vi "ADSR_RT.vi"() -> ()   [LabVIEW 2014]
uses:
  Controls/ADSR State.ctl
  <vilib>/myRIO/Instrument Drivers/Onboard IO/AudioOut Block/typedefs/AudioOut Block Reference.ctl
  <vilib>/myRIO/Common/Instrument Driver Framework/Utilities/typedefs/myRIO Generic Hardware Reference.ctl
  <vilib>/myRIO/Common/Instrument Driver Framework/Utilities/typedefs/Hardware Version Enum.ctl
  <vilib>/myRIO/Common/Instrument Driver Framework/Utilities/typedefs/myRIO v1.0 Reference.ctl
  <vilib>/myRIO/Common/Instrument Driver Framework/Utilities/typedefs/Generic FPGA Reference.ctl
  <vilib>/myRIO/Common/Instrument Driver Framework/myRIO v1.0/AudioOut Block/typedefs/AudioOut Block Channels List.ctl
  <vilib>/myRIO/Common/Instrument Driver Framework/myRIO v1.0/AudioOut Block/typedefs/AudioOut Block Channels Enum.ctl
  <vilib>/myRIO/Common/Instrument Driver Framework/Utilities/typedefs/Analog Scaling Constants.ctl
  <vilib>/userdefined/High Color/nirio_resource_hc.ctl
  <vilib>/myRIO/Common/Instrument Driver Framework/Utilities/vis/Is FPGA Ref Available.vi
  <vilib>/myRIO/Common/Instrument Driver Framework/myRIO v1.0/AudioOut Block/vis/myRIO v1.1 Open Throughput AudioOut (N Samples).vi
  <vilib>/myRIO/Instrument Drivers/Onboard IO/AudioOut Block/vis/Write.vi
  <vilib>/myRIO/Common/Instrument Driver Framework/Utilities/vis/Validate Channels.vi
  <vilib>/Utility/VariantDataType/GetNumericInfo.vi
  <vilib>/Utility/error.llb/Error Cluster From Error Code.vi
  <vilib>/myRIO/Common/Instrument Driver Framework/myRIO v1.0/myRIO v1.1 Open Throughput.vi
  <vilib>/myRIO/Common/Instrument Driver Framework/myRIO v1.0/AudioOut Block/vis/myRIO v1.0 Get Scaling Constants AudioOut Block.vi
  <vilib>/myRIO/Common/Instrument Driver Framework/myRIO v1.0/AudioOut Block/vis/myRIO v1.0 Reserve AudioOut Block.vi
  <vilib>/myRIO/Common/Instrument Driver Framework/myRIO v1.0/Resource Manager/vis/myRIO v1.0 Open Writing DMA.vi
  <vilib>/myRIO/Common/Instrument Driver Framework/myRIO v1.0/myRIO v1.0 Close.vi
  <vilib>/myRIO/Common/Instrument Driver Framework/myRIO v1.0/AudioOut Block/vis/myRIO v1.0 AudioOut Block Write.vi
  <vilib>/myRIO/Express VI/Onboard IO/AudioOut/AudioOut Express VI.xnode
  <vilib>/myRIO/Instrument Drivers/Onboard IO/AudioOut Block/vis/myRIO AudioOut N Samples Open.xnode
  <vilib>/myRIO/Instrument Drivers/Onboard IO/AudioOut Block/AudioOut Block.lvlib
  <vilib>/measure/NI_MABase.lvlib
panel:
  in  "Stop Button":bool
  in  "Activate 2":bool
  out "f":T1
  out "Gain Graph 2":dbl(graph)
  out "Gain2":dbl
  in  "Release":dbl=300.0
  in  "Sustain 2":dbl=300.0
  in  "Decay (ms) 2":dbl=300.0
  in  "Sustain  2":dbl=60.0
  in  "Max. Amplitude (V) 2":dbl(slide)=0.7993311036789298 scale=0.0..1.0
  in  "Attack (ms) 2":dbl=1000.0
  in  "sampling info":cluster{"Fs":dbl, "#s":dbl}={"Fs"=10000.0, "#s"=1000.0} {"Fs" format="%.2p"}
  in  "Pitch Frequency":dbl=2200.0 format="%#_13g"
  out "End of Idle":i32=1002
  out "End":bool
  out "error out":errorcluster
  out "Waveform Chart":dbl[](graph)
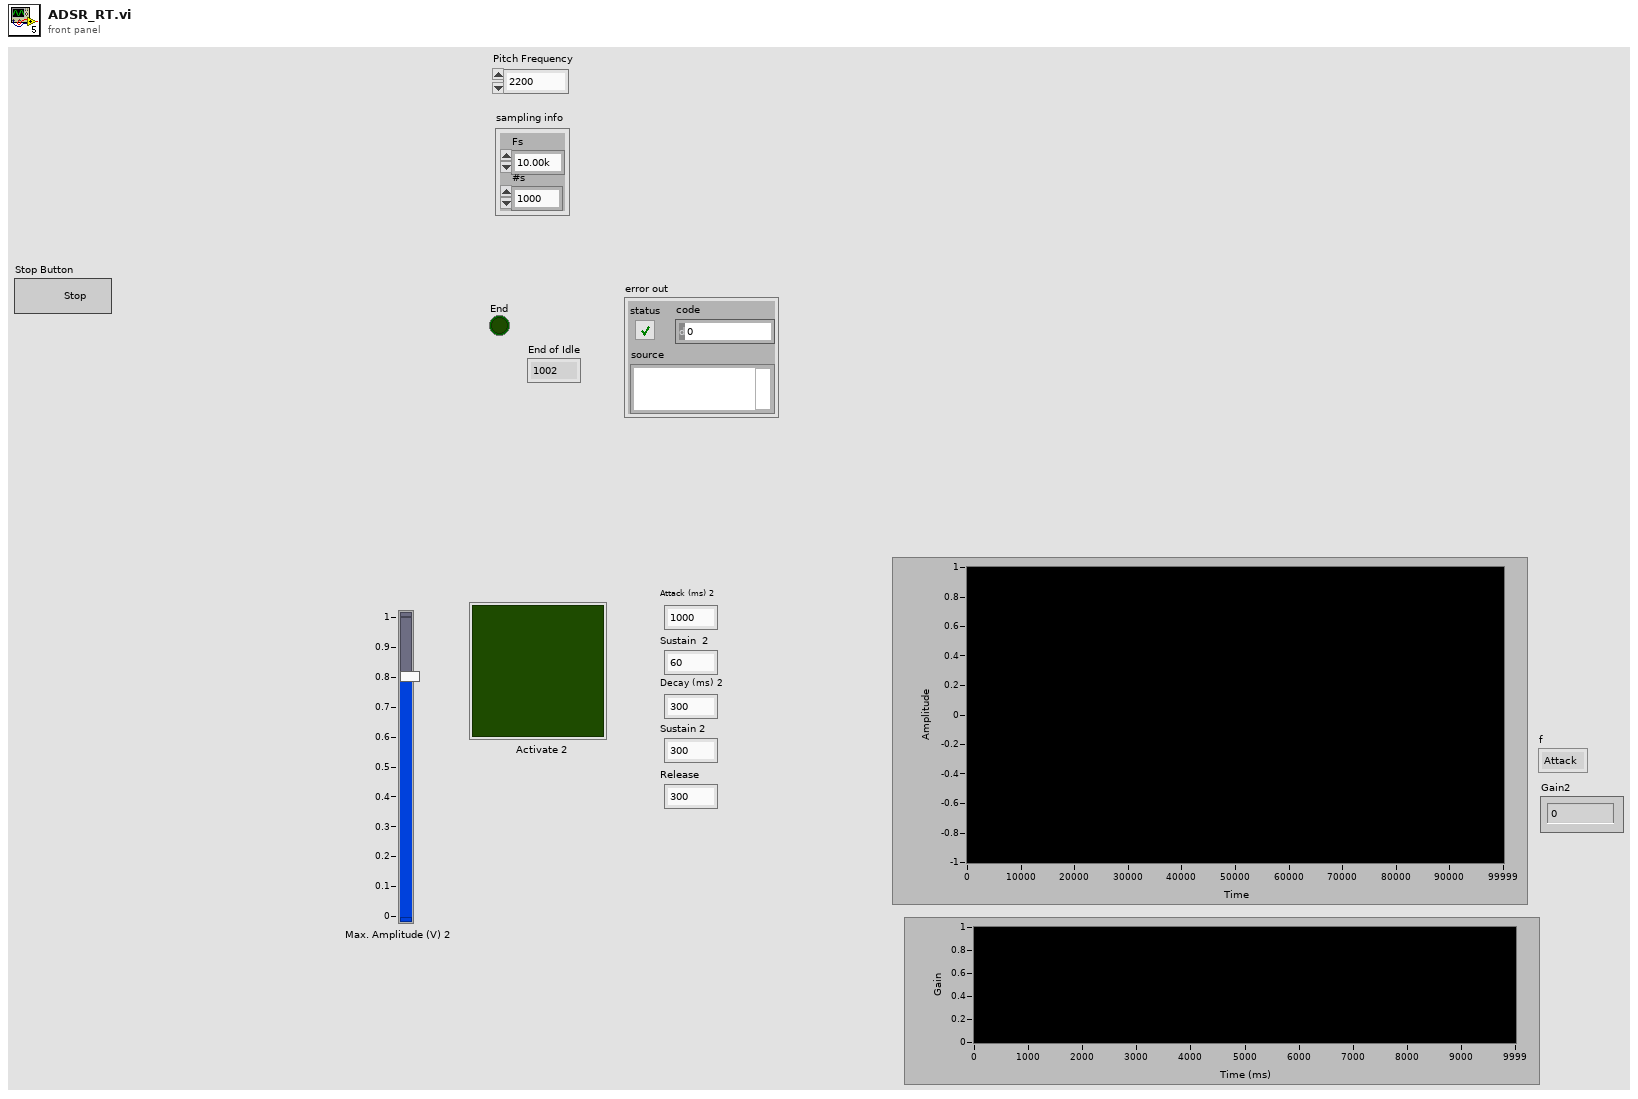
[diagram p1: front panel]
types:
  T1 = typedef "ADSR State.ctl" = enum16{"Attack", "Decay", "Sustain", "Release", "Idle"}
  T2 = typedef "AudioOut Block.lvlib/AudioOut Block Reference.ctl" = cluster{"myRIO Reference":T3, "AudioOut (N Samples) Channels List":T7, "AudioOut (N Samples) Scaling Constants List":T9[]}
  T3 = typedef "myRIO Generic Hardware Reference.ctl" = cluster{"myRIO Model":T4, "myRIO Hardware Reference":T5}
  T4 = typedef "Hardware Version Enum.ctl" = enum16{"Unknown", "myRIO-1900", "myRIO-1950"}
  T5 = typedef "myRIO v1.0 Reference.ctl" = cluster{"Generic FPGA Reference":T6, "Allow multiple opens":bool}
  T6 = typedef "Generic FPGA Reference.ctl" = refnum<k20>
  T7 = typedef "AudioOut Block Channels List.ctl" = T8[]
  T8 = typedef "AudioOut Block Channels Enum.ctl" = enum16{"Not Connected", "AudioOut/Left (N Samples)", "AudioOut/Right (N Samples)"}
  T9 = typedef "Analog Scaling Constants.ctl" = cluster{"LSB Weight (Volts)":dbl, "Offset (Volts)":dbl, "Signed?":bool}
  T10 = typedef "nirio_resource_hc.ctl" = tag
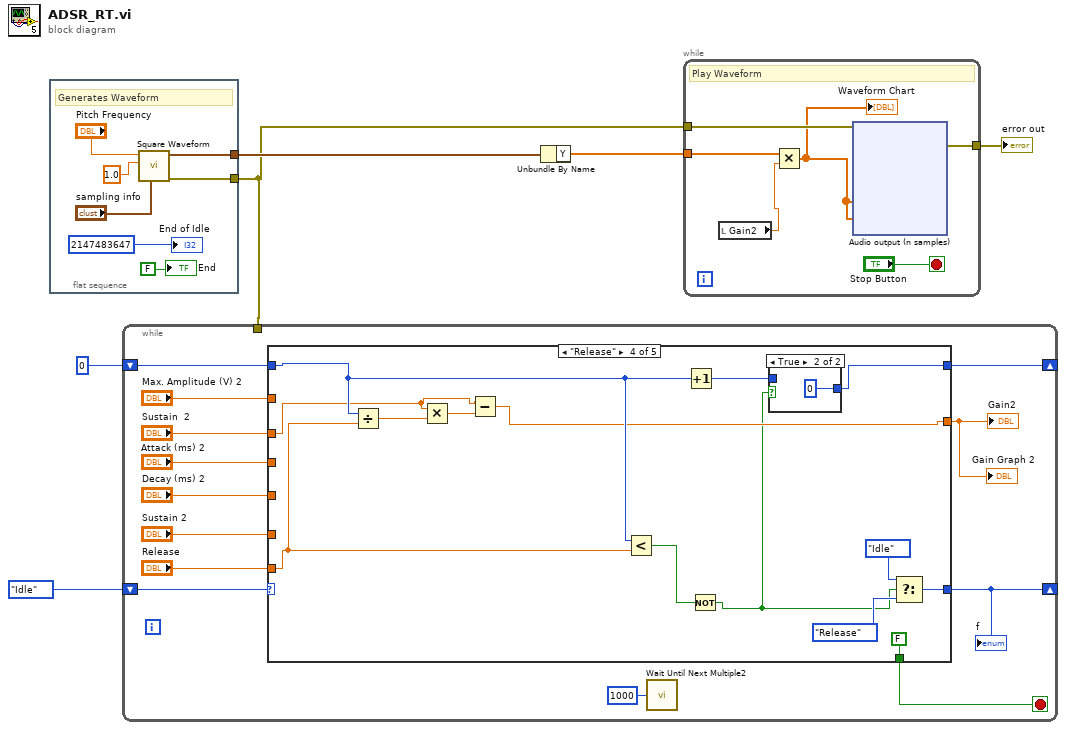
[diagram p0: block diagram]
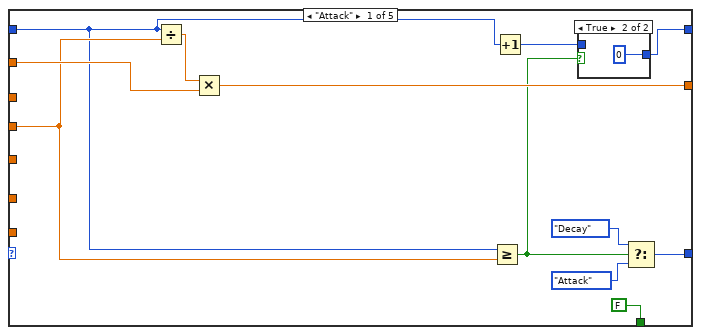
[diagram p2: hidden frame]
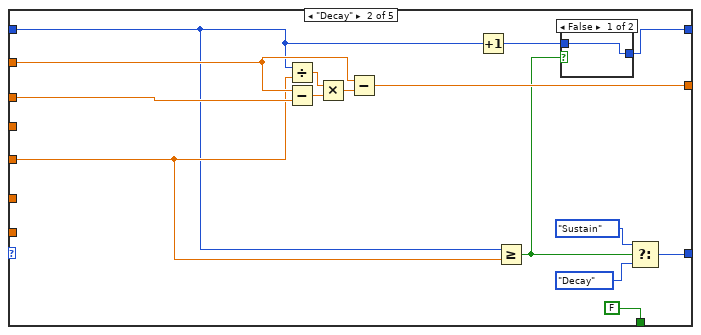
[diagram p4: hidden frame]
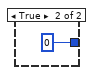
[diagram p5: hidden frame]
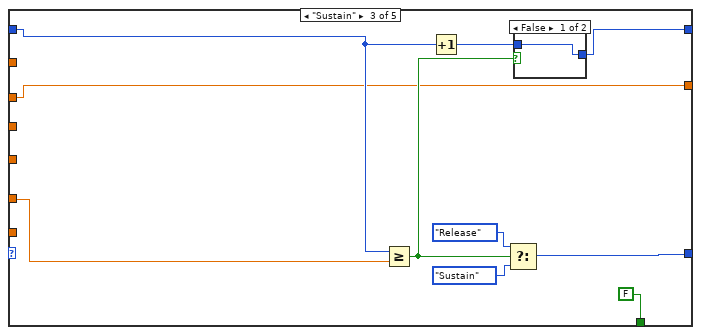
[diagram p6: hidden frame]
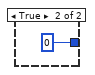
[diagram p7: hidden frame]
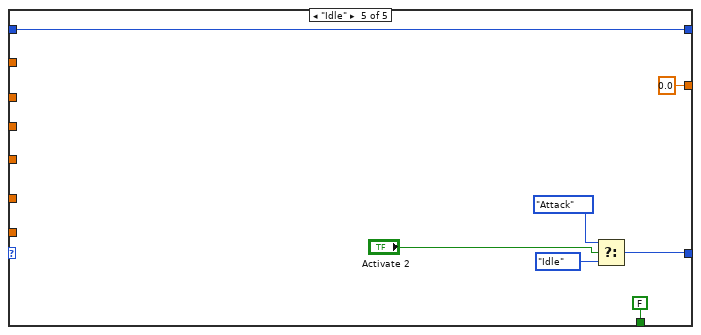
[diagram p9: hidden frame]
diagram:
  n1 = flat-sequence {
    tunnel: [w8] -> w4
    tunnel: [w9] -> w1
    frame #0 {
      # "Generates Waveform"
      n2 = call <vilib>:"Square Waveform.vi"("sampling info"="sampling info", "amplitude"=1.0, "frequency"="Pitch Frequency") -> ("error out"=w9:errorcluster, "signal out"=w8:waveform(dbl))  [unwired: 7 in]
      "End of Idle" <- 2147483647 ("End Sustain")
      "End" <- FALSE ("End")
    }
  }
  n3 = while {
    shift-right: [w19] -> _
    shift-left: ADSR_State."Idle" -> [w26]
    shift-right: [w16] -> _
    shift-left: 0 -> [w17]
    tunnel: w1 -> [_]
    stop <- w15 stop-if-true
    n4 = case shown="\"Release\"" w26 {
      tunnel: "Sustain  2" -> [_ w55 w59 w76 _]
      tunnel: "Max. Amplitude (V) 2" -> [w37 w52 _ _ _]
      tunnel: "Attack (ms) 2" -> [w32 _ _ _ _]
      tunnel: "Decay (ms) 2" -> [_ w46 _ _ _]
      tunnel: "Sustain 2" -> [_ _ w60 _ _]
      tunnel: "Release" -> [_ _ _ w79 _]
      tunnel: w17 -> [w30 w44 w61 w80 w90]
      tunnel: [w36 w50 w59 w75 0.0 ("Sustain (%) 2")] -> w14
      tunnel: [w33 w47 w63 w74 w89] -> w19
      tunnel: [w28 w42 w66 w82 w90] -> w16
      tunnel: [FALSE FALSE FALSE FALSE FALSE] -> w15
      frame "Attack" {
        n5 = Divide(x=w30, y=w32) -> (x/y=w38:dbl)
        n6 = Multiply(x=w38, y=w37) -> (x*y=w36:dbl)
        n7 = Greater Or Equal?(x=w30, y=w32) -> (x >= y?=w29:bool)
        n8 = Increment(x=w30) -> (x+1=w31:i32)
        n9 = case shown="True" w29 {
          tunnel: w31 -> [w39 _]
          tunnel: [w39 0] -> w28
          frame False {
          }
          frame True {
          }
        }
        n10 = Select(t=ADSR_State."Decay", s=w29, f=ADSR_State."Attack") -> (s? t:f=w33:T1)
      }
      frame "Decay" {
        n11 = Divide(x=w44, y=w46) -> (x/y=w54:dbl)
        n12 = Subtract(x=w52, y=w55) -> (x-y=w53:dbl)
        n13 = Multiply(x=w54, y=w53) -> (x*y=w51:dbl)
        n14 = Subtract(x=w52, y=w51) -> (x-y=w50:dbl)
        n15 = Increment(x=w44) -> (x+1=w43:i32)
        n16 = Greater Or Equal?(x=w44, y=w46) -> (x >= y?=w45:bool)
        n17 = case shown="False" w45 {
          tunnel: w43 -> [w56 _]
          tunnel: [w56 0] -> w42
          frame False {
          }
          frame True {
          }
        }
        n18 = Select(t=ADSR_State."Sustain", s=w45, f=ADSR_State."Decay") -> (s? t:f=w47:T1)
      }
      frame "Sustain" {
        n19 = Greater Or Equal?(x=w61, y=w60) -> (x >= y?=w62:bool)
        n20 = Increment(x=w61) -> (x+1=w67:i32)
        n21 = Select(t=ADSR_State."Release", s=w62, f=ADSR_State."Sustain") -> (s? t:f=w63:T1)
        n22 = case shown="False" w62 {
          tunnel: w67 -> [w68 _]
          tunnel: [w68 0] -> w66
          frame False {
          }
          frame True {
          }
        }
      }
      frame "Release" {
        n23 = Divide(x=w80, y=w79) -> (x/y=w78:dbl)
        n24 = Multiply(x=w76, y=w78) -> (x*y=w77:dbl)
        n25 = Subtract(x=w76, y=w77) -> (x-y=w75:dbl)
        n26 = Less?(x=w80, y=w79) -> (x < y?=w81:bool)
        n27 = Increment(x=w80) -> (x+1=w83:i32)
        n28 = Not(x=w81) -> (.not. x?=w71:bool)
        n29 = case shown="True" w71 {
          tunnel: w83 -> [w84 _]
          tunnel: [w84 0] -> w82
          frame False {
          }
          frame True {
          }
        }
        n30 = Select(t=ADSR_State."Idle", s=w71, f=ADSR_State."Release") -> (s? t:f=w74:T1)
      }
      frame "Idle" {
        n31 = Select(t=ADSR_State."Attack", s="Activate 2", f=ADSR_State."Idle") -> (s? t:f=w89:T1)
      }
    }
    "Gain2" <- w14
    "Gain Graph 2" <- w14
    "f" <- w19
    n32 = call "Wait Until Next Multiple2"("Count(uSec)"=u32 1000) -> ()  [unwired: 1 out]
  }
  n33 = Unbundle By Name(w4) -> ("Y"=w6:dbl[])
  n34 = while {
    tunnel: w6 -> [w96]
    tunnel: w1 -> [w97]
    tunnel: [w98] -> w5
    stop <- "Stop Button" stop-if-true
    # "Play Waveform"
    n35 = local read "Gain2"() -> (w94:dbl)
    n36 = Multiply(x=w96, y=w94) -> (x*y=w95:dbl[])
    "Waveform Chart" <- w95
    n37 = xnode "Audio output (n samples)"("AudioOut/Left (N Samples)"=w95, "AudioOut/Right (N Samples)"=w95, "error in (no error)"=w97) -> ("error out"=w98:errorcluster)
  }
  "error out" <- w5
